vi "Actor Core.vi"(8 "error in":errorcluster, 11 "GPU FFT Calculator in":refnum<class "GPU FFT Calculator.lvclass">) -> (0 "error out":errorcluster, 3 "Actor out":refnum<class "Actor.lvclass">)   [LabVIEW 2020, in "GPU FFT Calculator.lvlib" / "GPU FFT Calculator.lvclass"]
doc: "<p>(<strong>Filename</strong>: <span class=\"dnl\">Actor Framework.lvlib:Actor.lvclass:Actor Core.vi</span>)</p>\n<p>Receives messages to the actor, reacts to them, and initiates any error handling that may shut the actor down.</p>\n<p>Descendant classes may override this VI to append parallel tasks for the actor to complete while it handles messages. Overrides use the <a href=\"nihelplauncher://docs/csh?context=lvcore_glang_udclass\">Call Parent Class Method</a> node.</p>"
uses:
  GPU FFT Calculator.lvclass
  C:/Program Files/National Instruments/LabVIEW 2026/vi.lib/ActorFramework/Actor/Actor.lvclass
  <vilib>/ActorFramework/Actor/Actor.lvclass
  QMH Message.ctl
  <vilib>/Platform/TimedLoop/XDataNode/timing_clust.ctl
  <vilib>/Platform/TimedLoop/XDataNode/nitl_modes.ctl
  <vilib>/Platform/TimedLoop/XDataNode/wakeup.ctl
  GPU FFT Calculator.lvclass/GPU FFT Calculator.ctl
  GPU Device Message.ctl
  <vilib>/Natan Biesmans/G2CPU GPU and CPU HPC Toolkit/ArrayFire Driver/TypeDefs/backend.ctl
  GPU Calculation Message.ctl
  <vilib>/Natan Biesmans/G2CPU GPU and CPU HPC Toolkit/G2CPU Libraries/Async IO/DMA Manager/DMA Manager.lvclass
  <vilib>/Natan Biesmans/G2CPU GPU and CPU HPC Toolkit/G2CPU Libraries/Arrays/1DArray/s16/1D Array s16.lvclass
  C:/Program Files/National Instruments/LabVIEW 2026/vi.lib/Natan Biesmans/G2CPU GPU and CPU HPC Toolkit/G2CPU Libraries/Arrays/Array/Array Prototype.lvclass
  <vilib>/Natan Biesmans/G2CPU GPU and CPU HPC Toolkit/G2CPU Libraries/Arrays/1DArray/f32/1D Array f32.lvclass
  chart zoom.ctl
  GPU Metrics.ctl
  <vilib>/ActorFramework/Actor/Actor.lvclass/Actor.ctl
  <vilib>/ActorFramework/Message Enqueuer/Message Enqueuer.lvclass/Message Enqueuer.ctl
  GPU FFT Calculator Messages/Process Calculation Results Msg/Process Calculation Results Msg.lvclass/Process Calculation Results Msg.ctl
  <vilib>/Natan Biesmans/G2CPU GPU and CPU HPC Toolkit/G2CPU Libraries/Arrays/Array/Array Prototype.lvclass/Array Prototype.ctl
  8c2c1934-b7fc-4e70-9400-bf2723bb4974.vi
  dd08e257-5fd4-41c3-ab12-3278198c71ec.vi
  1389a678-718d-4937-8c80-96463c139bed.vi
  ec50676d-beb5-455b-a2b4-c30064f406c8.vi
  7e026b22-0010-41a1-b2bb-e8234edaae8f.vi
  <vilib>/ActorFramework/Message Enqueuer/Init from Existing Queue.vi
  <vilib>/Natan Biesmans/G2CPU GPU and CPU HPC Toolkit/ArrayFire Driver/VIs/Run as Multi Device.vi
  <vilib>/ActorFramework/Message Enqueuer/Enqueue.vi
  dd08e257-5fd4-41c3-ab12-3278198c71ec.vi/67bb9abe-6be7-467c-be3d-dc59a1f5a88b.vi
  dd08e257-5fd4-41c3-ab12-3278198c71ec.vi/bc198a8f-250c-4fb0-95cf-f9e16e559b40.vi
  dd08e257-5fd4-41c3-ab12-3278198c71ec.vi/206e65cf-1cd8-4fd2-b98d-94b74801007d.vi
  <vilib>/Natan Biesmans/G2CPU GPU and CPU HPC Toolkit/G2CPU Libraries/Arrays/Array/G2CPU Get Array Pointer.vi
  1389a678-718d-4937-8c80-96463c139bed.vi/6197f869-f6d4-49b3-9b2c-cc979b422c2e.vi
  1389a678-718d-4937-8c80-96463c139bed.vi/a7e86dbb-b4c0-485c-89c5-522e60ee265c.vi
  ec50676d-beb5-455b-a2b4-c30064f406c8.vi/ff52a514-0e94-4685-9782-cee11f20a7e4.vi
  ec50676d-beb5-455b-a2b4-c30064f406c8.vi/09f95493-deb6-40ba-ba08-e63bad1f3c71.vi
  7e026b22-0010-41a1-b2bb-e8234edaae8f.vi/7467a0f1-0650-4e63-b635-b3d2b2ec9a4e.vi
  7e026b22-0010-41a1-b2bb-e8234edaae8f.vi/8ee11bc3-5ef5-497e-97f0-8db2b3aaa149.vi
  7e026b22-0010-41a1-b2bb-e8234edaae8f.vi/c7af9698-5e3c-4e11-95da-3024075b67d2.vi
  1389a678-718d-4937-8c80-96463c139bed.vi/6197f869-f6d4-49b3-9b2c-cc979b422c2e.vi/3e802c67-fb96-46a3-ae13-4994a8508b4f.vi
  1389a678-718d-4937-8c80-96463c139bed.vi/6197f869-f6d4-49b3-9b2c-cc979b422c2e.vi/5a50fc67-79e7-4972-80c2-92243cd53dd4.vi
  1389a678-718d-4937-8c80-96463c139bed.vi/6197f869-f6d4-49b3-9b2c-cc979b422c2e.vi/1c928fc9-710a-40e7-8c4f-08a1069452ae.vi
  1389a678-718d-4937-8c80-96463c139bed.vi/a7e86dbb-b4c0-485c-89c5-522e60ee265c.vi/730f6c57-5c0b-4ee9-b61e-75067b25222b.vi
  1389a678-718d-4937-8c80-96463c139bed.vi/a7e86dbb-b4c0-485c-89c5-522e60ee265c.vi/096b8799-7810-404e-baca-ba9279cec4bd.vi
  1389a678-718d-4937-8c80-96463c139bed.vi/a7e86dbb-b4c0-485c-89c5-522e60ee265c.vi/0f1a5a47-bcc5-4796-ac31-8dfcfbc0d7d1.vi
  1389a678-718d-4937-8c80-96463c139bed.vi/a7e86dbb-b4c0-485c-89c5-522e60ee265c.vi/89f12e17-3330-4b72-ad8f-8dd636660732.vi
  1389a678-718d-4937-8c80-96463c139bed.vi/6197f869-f6d4-49b3-9b2c-cc979b422c2e.vi/3e802c67-fb96-46a3-ae13-4994a8508b4f.vi/1b7cf390-2ae0-48f3-9bce-03c57eed6ee8.vi
  GPU FFT Calculator Messages/Process Calculation Results Msg/Process Calculation Results Msg.lvclass
  C:/Program Files/National Instruments/LabVIEW 2026/vi.lib/ActorFramework/Message/Message.lvclass
  <vilib>/Natan Biesmans/G2CPU GPU and CPU HPC Toolkit/G2CPU Libraries/Arrays/1DArray/c32/1D Array c32.lvclass
  <vilib>/Natan Biesmans/G2CPU GPU and CPU HPC Toolkit/G2CPU Libraries/Arrays/2DArray/c32/2D Array c32.lvclass
  <vilib>/Natan Biesmans/G2CPU GPU and CPU HPC Toolkit/G2CPU Libraries/Arrays/2DArray/f32/2D Array f32.lvclass
  <vilib>/Natan Biesmans/G2CPU GPU and CPU HPC Toolkit/ArrayFire Driver/subvi/Error Converter (ErrCode or Status).vi
  <vilib>/Natan Biesmans/G2CPU GPU and CPU HPC Toolkit/G2CPU Libraries/Arrays/Array/G2CPU Set Array Pointer.vi
  <vilib>/Natan Biesmans/G2CPU GPU and CPU HPC Toolkit/G2CPU Libraries/Arrays/SubVI/is 2D.vi
  <vilib>/Natan Biesmans/G2CPU GPU and CPU HPC Toolkit/ArrayFire Driver/VIs/mul.vi
  <vilib>/Natan Biesmans/G2CPU GPU and CPU HPC Toolkit/ArrayFire Driver/VIs/fft inplace.vi
  <vilib>/Natan Biesmans/G2CPU GPU and CPU HPC Toolkit/ArrayFire Driver/VIs/flat.vi
  <vilib>/Natan Biesmans/G2CPU GPU and CPU HPC Toolkit/G2CPU Libraries/Manage Environment/G2CPU Get Backend.vi
  <vilib>/Utility/error.llb/Error Cluster From Error Code.vi
  <vilib>/Natan Biesmans/G2CPU GPU and CPU HPC Toolkit/G2CPU Libraries/Async IO/CUDA Context FGV.vi
  <vilib>/Natan Biesmans/G2CPU GPU and CPU HPC Toolkit/ArrayFire Driver/VIs/copy array.vi
  <vilib>/ActorFramework/Message Priority Queue/Priority Enqueue.vi
  Calculation Worker/Calculation Worker/Calculation Worker.lvclass
  <vilib>/platform/TimedLoop/XDataNode/XDataNode.xnode
  <vilib>/Natan Biesmans/G2CPU GPU and CPU HPC Toolkit/G2CPU Libraries/Arrays/DataTypes/c32/c32.lvclass
  <vilib>/Natan Biesmans/G2CPU GPU and CPU HPC Toolkit/G2CPU Libraries/Arrays/2DArray/2D Array Prototype.lvclass
  <vilib>/Natan Biesmans/G2CPU GPU and CPU HPC Toolkit/G2CPU Libraries/Arrays/Array/Array Prototype.lvclass
  <vilib>/Natan Biesmans/G2CPU GPU and CPU HPC Toolkit/G2CPU Libraries/Arrays/1DArray/1D Array Prototype.lvclass
  <vilib>/Natan Biesmans/G2CPU GPU and CPU HPC Toolkit/G2CPU Libraries/Arrays/DataTypes/f32/f32.lvclass
  <vilib>/ActorFramework/Message Enqueuer/Message Enqueuer.lvclass
  <vilib>/Natan Biesmans/G2CPU GPU and CPU HPC Toolkit/G2CPU Libraries/Manage Environment/G2CPU Manage Environment.lvlib
  <vilib>/Platform/TimedLoop/XDataNode/XDNodeRunTimeDep.lvlib
  <vilib>/Natan Biesmans/G2CPU GPU and CPU HPC Toolkit/ArrayFire Driver/AF.lvlib
  Simple UI/Simple UI/Simple UI.lvclass
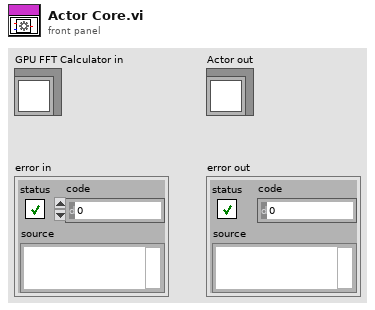
[diagram p1: front panel]
types:
  T1 = typedef "GPU FFT Calculator.lvlib/GPU FFT Calculator.lvclass/QMH Message.ctl" = cluster{"Command":string, "Data":variant}
  T2 = typedef "XDNodeRunTimeDep.lvlib/timing_clust.ctl" = cluster{"Expected End [f-1]":u64, "Actual End [f-1]":u64, "Finished Late? [f-1]":bool, "Expected End [i-1]":u64, "Actual End [i-1]":u64, "Finished Late? [i-1]":bool, "Expected Start [i]":u64, "Actual Start [i]":u64, "Expected Start [f]":u64, "Actual Start [f]":u64, "Source Name":string, "Structure Name":string, "Period":i64, "Deadline":i64, "Offset":i64, "Start":i64, "Priority":i32, "Timeout":i32, "Mode":T3, "Wakeup Reason":T4, "Error":errorcluster, "Source Type":string, "Secondary Source Type":string, "Global End Time":u64, "Global Start Time":u64, "Frame Duration":u64, "Iteration Duration":u64, "Assigned CPU":i32, "I/O Scan Engine Mode":u32}
  T3 = typedef "XDNodeRunTimeDep.lvlib/nitl_modes.ctl" = enum32{"No Change", "Process missed periods, maintain original phase", "Discard missed periods, maintain original phase", "Process missed periods, ignore original phase", "Discard missed periods, ignore original phase"}
  T4 = typedef "XDNodeRunTimeDep.lvlib/wakeup.ctl" = enum32{"Normal", "Aborted", "Asynchronous wakeup", "Timing source error", "Timed loop error", "Timeout"}
  T5 = typedef "GPU FFT Calculator.lvlib/GPU FFT Calculator.lvclass/GPU Device Message.ctl" = cluster{"Backend":T6, "Device ID":i32}
  T6 = typedef "AF.lvlib/backend.ctl" = u32
  T7 = typedef "GPU FFT Calculator.lvlib/GPU FFT Calculator.lvclass/GPU Calculation Message.ctl" = cluster{"FFT Size":u64, "Batch Size":u64, "dt":dbl, "Result Buffer":refnum<data-value>, "gain":dbl, "Zoom Parameters":T8, "Upload DMA Manager":refnum<class "DMA Manager.lvclass">, "Data Buffer":refnum<data-value>, "Data Buffer GPU":refnum<class "1D Array s16.lvclass">, "GPU Metrics":T9, "df":dbl, "f0":dbl, "Zoomed Size":u64, "Result Buffer GPU":refnum<class "1D Array f32.lvclass">, "Start Time":dbl, "Batch Index":i32, "Amount of Batches":i32, "Download DMA Manager":refnum<class "DMA Manager.lvclass">}
  T8 = typedef "Simple UI.lvlib/Simple UI.lvclass/chart zoom.ctl" = cluster{"Override":bool, "f0: ":dbl, "fwidth: ":dbl}
  T9 = typedef "GPU FFT Calculator.lvlib/GPU FFT Calculator.lvclass/GPU Metrics.ctl" = cluster{"Upload Time":dbl, "Algorithm Processing Time":dbl, "Single Trace Size":u64}
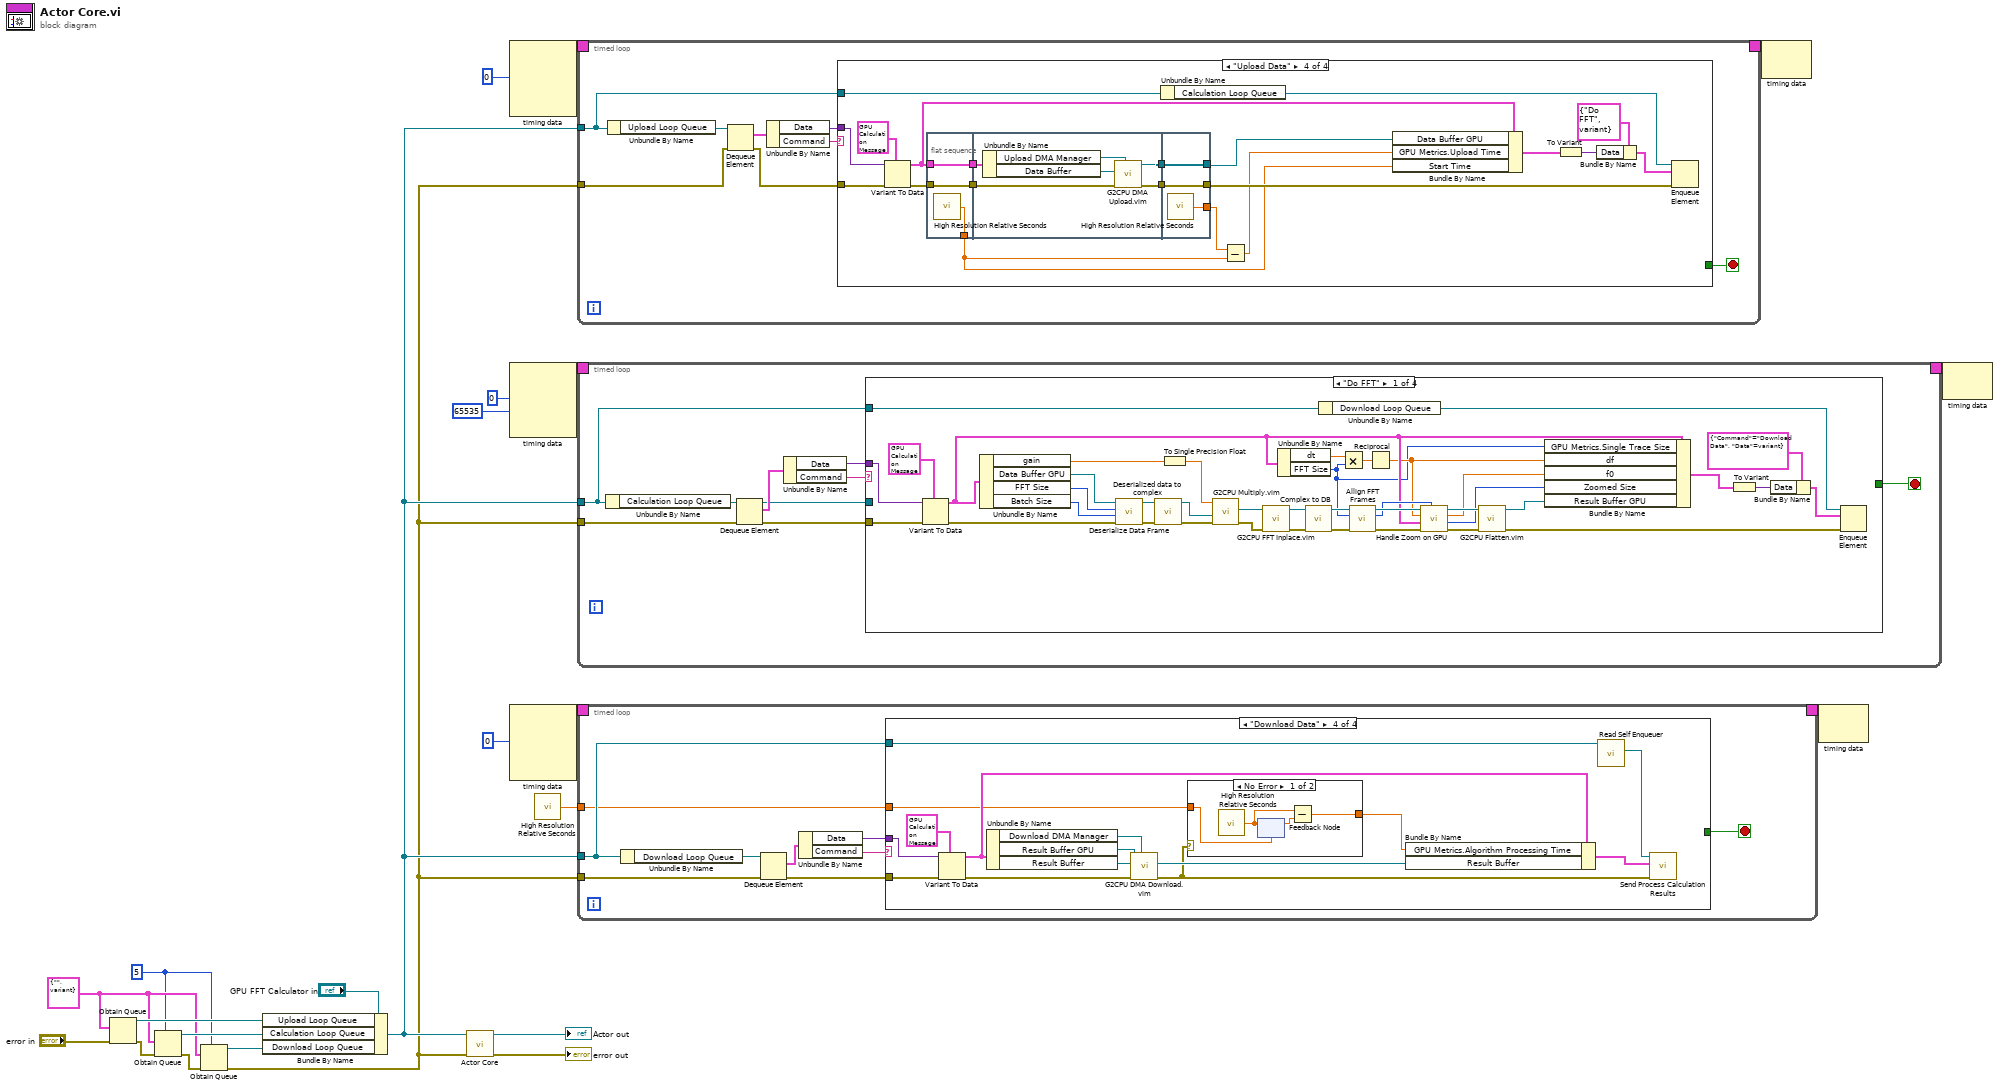
[diagram p0: block diagram]
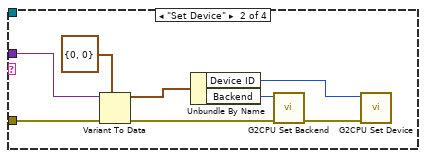
[diagram p3: hidden frame]
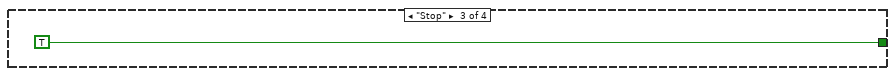
[diagram p4: hidden frame]
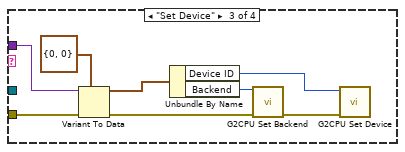
[diagram p6: hidden frame]
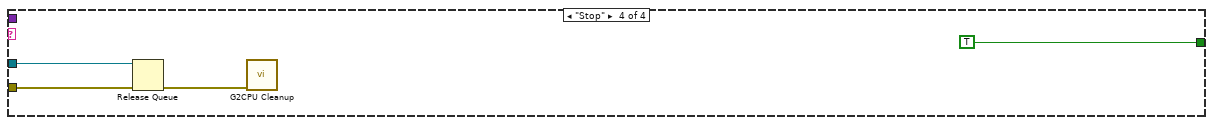
[diagram p7: hidden frame]
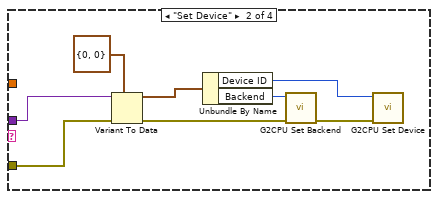
[diagram p9: hidden frame]
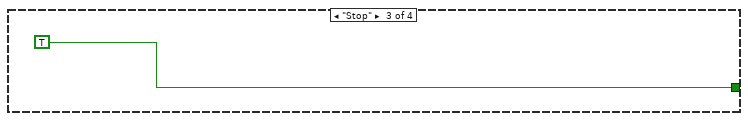
[diagram p10: hidden frame]
diagram:
  w2 = 5 ("max queue size (-1, unlimited)")
  w5 = T1 {"Command"="", "Data"=variant}
  n1 = Obtain Queue(element data type=w5, error in (no error)="error in") -> (queue out=w17:refnum<queue>, error out=w9:errorcluster)  [unwired: 3 in, 1 out]
  n2 = Obtain Queue(max queue size (-1, unlimited)=w2, element data type=w5, error in (no error)=w9) -> (queue out=w8:refnum<queue>, error out=w7:errorcluster)  [unwired: 2 in, 1 out]
  n3 = Obtain Queue(max queue size (-1, unlimited)=w2, element data type=w5, error in (no error)=w7) -> (queue out=w6:refnum<queue>, error out=w4:errorcluster)  [unwired: 2 in, 1 out]
  n4 = Bundle By Name(cluster="GPU FFT Calculator in", "Upload Loop Queue"=w17, "Calculation Loop Queue"=w8, "Download Loop Queue"=w6) -> (w15:refnum<class "GPU FFT Calculator.lvclass">)
  n5 = call-parent "Actor Core.vi"("error in"=w4, "Actor in"=w15) -> ("error out"=→"error out":errorcluster, "Actor out"=→"Actor out":refnum<class "Actor.lvclass">)  [unwired: 8 in]
  n6 = node-c288(i64 0 ("Period")) -> (w14:T2)  [unwired: 3 in]
  n7 = node-c288(i64 0 ("Period"), 65535 ("Priority")) -> (w22:T2)  [unwired: 2 in]
  n8 = node-c288(i64 0 ("Period")) -> (w11:T2)  [unwired: 3 in]
  n9 = call <vilib>:"High Resolution Relative Seconds.vi"() -> ("relative seconds"=w1:dbl)
  n10 = timed-loop {
    timing: w14 -> [_]
    timing-out: [_] -> w13
    tunnel: w15 -> [w25]
    tunnel: w4 -> [w28]
    stop <- w26 stop-if-true
    n11 = Unbundle By Name(w25) -> ("Upload Loop Queue"=w32:refnum<queue>)
    n12 = Dequeue Element(queue=w32, error in (no error)=w28) -> (element=w31:T1, error out=w27:errorcluster)  [unwired: 1 in, 2 out]
    n13 = Unbundle By Name(w31) -> ("Data"=w29:variant, "Command"=w30:string)
    n14 = case shown="\"Upload Data\"" w30 {
      tunnel: w29 -> [_ w34 _ w58]
      tunnel: w27 -> [_ w33 _ w59]
      tunnel: [_ _ TRUE _] -> w26
      tunnel: w25 -> [_ _ _ w51]
      frame "False", Default {
      }
      frame "Set Device" {
        n15 = Variant To Data(error in=w33, type=T5 {"Backend"=0, "Device ID"=0}, Variant=w34) -> (data=w38:T5, error out=w37:errorcluster)
        n16 = Unbundle By Name(w38) -> ("Device ID"=w40:i32, "Backend"=w39:T6)
        n17 = call <vilib>:"G2CPU Set Backend.vi"("error in (no error)"=w37, "Backend"=w39) -> ("error out"=w35:errorcluster)  [unwired: 9 in]
        n18 = call <vilib>:"G2CPU Set Device.vi"("error in (no error)"=w35, "Device ID"=w40) -> ()  [unwired: 9 in, 1 out]
      }
      frame "Stop" {
      }
      frame "Upload Data" {
        n19 = Variant To Data(error in=w59, type=T7 {"FFT Size"=0, "Batch Size"=0, "dt"=0.0, "Result Buffer"=refnum, "gain"=0.0, "Zoom Parameters"={"Override"=FALSE, "f0: "=0.0, "fwidth: "=0.0}, "Upload DMA Manager"=refnum, "Data Buffer"=refnum, "Data Buffer GPU"=refnum, "GPU Metrics"={"Upload Time"=0.0, "Algorithm Processing Time"=0.0, "Single Trace Size"=0}, "df"=0.0, "f0"=0.0, "Zoomed Size"=0, "Result Buffer GPU"=refnum, "Start Time"=0.0, "Batch Index"=0, "Amount of Batches"=0, "Download DMA Manager"=refnum} ("element"), Variant=w58) -> (data=w49:T7, error out=w60:errorcluster)
        n20 = flat-sequence {
          tunnel: w60 -> [w63]
          tunnel: w49 -> [w64]
          tunnel: [w64] -> w55
          tunnel: [w63] -> w54
          tunnel: [w62] -> w42
          tunnel: [w66] -> w57
          tunnel: [w65] -> w56
          tunnel: w55 -> [w70]
          tunnel: w54 -> [w68]
          tunnel: [w72] -> w52
          tunnel: [w73] -> w48
          tunnel: w57 -> [w73]
          tunnel: w56 -> [w72]
          tunnel: [w71] -> w53
          frame #0 {
            n21 = call <vilib>:"High Resolution Relative Seconds.vi"() -> ("relative seconds"=w62:dbl)
          }
          frame #1 {
            n22 = Unbundle By Name(w70) -> ("Upload DMA Manager"=w69:refnum<class "DMA Manager.lvclass">, "Data Buffer"=w67:refnum<data-value>)
            n23 = call "G2CPU DMA Upload.vim"("DMA Manager"=w69, "error in (no error)"=w68, "Data In"=w67) -> ("error out"=w65:errorcluster, "Array out"=w66:refnum<class "1D Array s16.lvclass">)  [unwired: 6 in, 1 out]
          }
          frame #2 {
            n24 = call <vilib>:"High Resolution Relative Seconds.vi"() -> ("relative seconds"=w71:dbl)
          }
        }
        n25 = Unbundle By Name(w51) -> ("Calculation Loop Queue"=w50:refnum<queue>)
        n26 = Subtract(x=w53, y=w42) -> (x-y=w47:dbl)
        n27 = Bundle By Name(cluster=w49, "Data Buffer GPU"=w48, "GPU Metrics.Upload Time"=w47, "Start Time"=w42) -> (w46:T7)
        n28 = To Variant(anything=w46) -> (Variant=w44:variant)
        n29 = Bundle By Name(cluster=T1 {"Command"="Do FFT", "Data"=variant} ("element"), "Data"=w44) -> (w43:T1)
        n30 = Enqueue Element(queue=w50, element=w43, error in (no error)=w52) -> ()  [unwired: 1 in, 3 out]
      }
    }
  }
  n31 = timed-loop {
    timing: w22 -> [_]
    timing-out: [_] -> w21
    tunnel: w15 -> [w77]
    tunnel: w4 -> [w83]
    stop <- w79 stop-if-true
    n32 = Unbundle By Name(w77) -> ("Calculation Loop Queue"=w84:refnum<queue>)
    n33 = Dequeue Element(queue=w84, error in (no error)=w83) -> (queue out=w76:refnum<queue>, element=w78:T1, error out=w81:errorcluster)  [unwired: 1 in, 1 out]
    n34 = Unbundle By Name(w78) -> ("Data"=w80:variant, "Command"=w82:string)
    n35 = case shown="\"Do FFT\"" w82 {
      tunnel: w81 -> [w123 _ w129 w133]
      tunnel: w80 -> [w122 _ w127 _]
      tunnel: [_ _ _ TRUE] -> w79
      tunnel: w76 -> [_ _ _ w134]
      tunnel: w77 -> [w97 _ _ _]
      frame "Do FFT" {
        n36 = Variant To Data(error in=w123, type=T7 {"FFT Size"=0, "Batch Size"=0, "dt"=0.0, "Result Buffer"=refnum, "gain"=0.0, "Zoom Parameters"={"Override"=FALSE, "f0: "=0.0, "fwidth: "=0.0}, "Upload DMA Manager"=refnum, "Data Buffer"=refnum, "Data Buffer GPU"=refnum, "GPU Metrics"={"Upload Time"=0.0, "Algorithm Processing Time"=0.0, "Single Trace Size"=0}, "df"=0.0, "f0"=0.0, "Zoomed Size"=0, "Result Buffer GPU"=refnum, "Start Time"=0.0, "Batch Index"=0, "Amount of Batches"=0, "Download DMA Manager"=refnum} ("element"), Variant=w122) -> (data=w92:T7, error out=w120:errorcluster)
        n37 = Unbundle By Name(w92) -> ("gain"=w100:dbl, "Data Buffer GPU"=w101:refnum<class "1D Array s16.lvclass">, "FFT Size"=w117:u64, "Batch Size"=w116:u64)
        n38 = call "Deserialize Data Frame.vi"("error in (no error)"=w120, "Batch Size"=w116, "FFT Size"=w117, "Serial Data In"=w101) -> ("error out"=w115:errorcluster, "Deserialized Data Out"=w114:refnum<class "3D Array s16.lvclass">)  [unwired: 6 in]
        n39 = call "Deserialized data to complex.vi"("error in (no error)"=w115, "Deserialized Data In"=w114) -> ("error out"=w113:errorcluster, "Complex Data Out"=w112:refnum<class "2D Array c32.lvclass">)  [unwired: 8 in]
        n40 = To Single Precision Float(number=w100) -> (single precision float=w109:sgl)
        n41 = call "G2CPU Multiply.vim"("error in (no error)"=w113, "Array rhs"=w112, "Array lhs"=w109) -> ("error out"=w107:errorcluster, "Array Result"=w108:refnum<class "2D Array c32.lvclass">)  [unwired: 7 in]
        n42 = call "G2CPU FFT Inplace.vim"("error in (no error)"=w107, "Array Signal"=w108) -> ("error out"=w111:errorcluster, "Array out"=w110:refnum<class "2D Array c32.lvclass">)  [unwired: 8 in]
        n43 = Unbundle By Name(w92) -> ("dt"=w118:dbl, "FFT Size"=w85:u64)
        n44 = call "Complex to DB.vi"("error in (no error)"=w111, "Complex Data In"=w110) -> ("error out"=w102:errorcluster, "Amplitude dB Out"=w106:refnum<class "2D Array f32.lvclass">)  [unwired: 8 in]
        n45 = Unbundle By Name(w97) -> ("Download Loop Queue"=w93:refnum<queue>)
        n46 = Multiply(x=w118, y=w85) -> (x*y=w119:dbl)
        n47 = call "Allign FFT Frames.vi"("error in (no error)"=w102, "FFT Size"=w85, "Unalligned FFT Amplitudes"=w106) -> ("error out"=w104:errorcluster, "FFT Size / 2"=w103:u64, "Unalligned FFT Amplitudes"=w105:refnum<class "2D Array f32.lvclass">)  [unwired: 6 in]
        n48 = Reciprocal(x=w119) -> (1/x=w91:dbl)
        n49 = call "Handle Zoom on GPU.vi"("FFT Size / 2 in"=w103, "error in (no error)"=w104, "element"=w92, "df"=w91, "Unzoomed Data In"=w105) -> ("error out"=w98:errorcluster, "Zoomed Size"=w89:u64, "f0:"=w90:dbl, "Zoomed Data Out"=w99:refnum<class "2D Array f32.lvclass">)  [unwired: 3 in]
        n50 = call "G2CPU Flatten.vim"("error in (no error)"=w98, "Array In"=w99) -> ("error out"=w86:errorcluster, "Array out"=w88:refnum<class "1D Array f32.lvclass">)  [unwired: 8 in]
        n51 = Bundle By Name(cluster=w92, "GPU Metrics.Single Trace Size"=w85, "df"=w91, "f0"=w90, "Zoomed Size"=w89, "Result Buffer GPU"=w88) -> (w87:T7)
        n52 = To Variant(anything=w87) -> (Variant=w95:variant)
        n53 = Bundle By Name(cluster=T1 {"Command"="Download Data", "Data"=variant} ("element"), "Data"=w95) -> (w96:T1)
        n54 = Enqueue Element(queue=w93, element=w96, error in (no error)=w86) -> ()  [unwired: 1 in, 3 out]
      }
      frame Default {
      }
      frame "Set Device" {
        n55 = Variant To Data(error in=w129, type=T5 {"Backend"=0, "Device ID"=0}, Variant=w127) -> (data=w126:T5, error out=w128:errorcluster)
        n56 = Unbundle By Name(w126) -> ("Device ID"=w124:i32, "Backend"=w125:T6)
        n57 = call <vilib>:"G2CPU Set Backend.vi"("error in (no error)"=w128, "Backend"=w125) -> ("error out"=w131:errorcluster)  [unwired: 9 in]
        n58 = call <vilib>:"G2CPU Set Device.vi"("error in (no error)"=w131, "Device ID"=w124) -> ()  [unwired: 9 in, 1 out]
      }
      frame "Stop" {
        n59 = Release Queue(queue=w134, error in (no error)=w133) -> (error out=w132:errorcluster)  [unwired: 1 in, 2 out]
        n60 = call <vilib>:"G2CPU Cleanup.vi"("error in (no error)"=w132) -> ()  [unwired: 10 in, 1 out]
      }
    }
  }
  n61 = timed-loop {
    timing: w11 -> [_]
    timing-out: [_] -> w10
    tunnel: w15 -> [w139]
    tunnel: w4 -> [w141]
    tunnel: w1 -> [w138]
    stop <- w140 stop-if-true
    n62 = Unbundle By Name(w139) -> ("Download Loop Queue"=w142:refnum<queue>)
    n63 = Dequeue Element(queue=w142, error in (no error)=w141) -> (element=w143:T1, error out=w146:errorcluster)  [unwired: 1 in, 2 out]
    n64 = Unbundle By Name(w143) -> ("Data"=w145:variant, "Command"=w144:string)
    n65 = case shown="\"Download Data\"" w144 {
      tunnel: w145 -> [_ w148 _ w164]
      tunnel: w146 -> [_ w147 _ w165]
      tunnel: [_ _ TRUE _] -> w140
      tunnel: w139 -> [_ _ _ w166]
      tunnel: w138 -> [_ _ _ w157]
      frame "False", Default {
      }
      frame "Set Device" {
        n66 = Variant To Data(error in=w147, type=T5 {"Backend"=0, "Device ID"=0}, Variant=w148) -> (data=w152:T5, error out=w151:errorcluster)
        n67 = Unbundle By Name(w152) -> ("Device ID"=w154:i32, "Backend"=w153:T6)
        n68 = call <vilib>:"G2CPU Set Backend.vi"("error in (no error)"=w151, "Backend"=w153) -> ("error out"=w149:errorcluster)  [unwired: 9 in]
        n69 = call <vilib>:"G2CPU Set Device.vi"("error in (no error)"=w149, "Device ID"=w154) -> ()  [unwired: 9 in, 1 out]
      }
      frame "Stop" {
      }
      frame "Download Data" {
        n70 = Variant To Data(error in=w165, type=T7 {"FFT Size"=0, "Batch Size"=0, "dt"=0.0, "Result Buffer"=refnum, "gain"=0.0, "Zoom Parameters"={"Override"=FALSE, "f0: "=0.0, "fwidth: "=0.0}, "Upload DMA Manager"=refnum, "Data Buffer"=refnum, "Data Buffer GPU"=refnum, "GPU Metrics"={"Upload Time"=0.0, "Algorithm Processing Time"=0.0, "Single Trace Size"=0}, "df"=0.0, "f0"=0.0, "Zoomed Size"=0, "Result Buffer GPU"=refnum, "Start Time"=0.0, "Batch Index"=0, "Amount of Batches"=0, "Download DMA Manager"=refnum} ("element"), Variant=w164) -> (data=w162:T7, error out=w169:errorcluster)
        n71 = Unbundle By Name(w162) -> ("Download DMA Manager"=w160:refnum<class "DMA Manager.lvclass">, "Result Buffer GPU"=w159:refnum<class "1D Array f32.lvclass">, "Result Buffer"=w161:refnum<data-value>)
        n72 = call "G2CPU DMA Download.vim"("DMA Manager"=w160, "error in (no error)"=w169, "Data In"=w161, "GPU CUDA Array In"=w159) -> ("error out"=w158:errorcluster, "Data Out"=w163:refnum<data-value>)  [unwired: 5 in, 1 out]
        n73 = case shown="No Error" w158 {
          tunnel: w157 -> [w171 _]
          tunnel: [w172 _] -> w156
          frame No Error {
            n74 = call <vilib>:"High Resolution Relative Seconds.vi"() -> ("relative seconds"=w173:dbl)
            n75 = feedback-in #1(w173) -> ()
            n76 = feedback #1(w171) -> (w174:dbl)
            n77 = Subtract(x=w173, y=w174) -> (x-y=w172:dbl)
          }
          frame Error {
          }
        }
        n78 = Bundle By Name(cluster=w162, "GPU Metrics.Algorithm Processing Time"=w156, "Result Buffer"=w163) -> (w168:T7)
        n79 = call <vilib>:"Read Self Enqueuer.vi"("Actor"=w166) -> ("Self Enqueuer"=w167:refnum<class "Message Enqueuer.lvclass">)  [unwired: 10 in]
        n80 = call "Send Process Calculation Results.vi"("error in (no error)"=w158, "GPU Calculation Results"=w168, "Message Enqueuer"=w167) -> ()  [unwired: 7 in, 2 out]
      }
    }
  }
  n81 = node-c288(w13) -> ()  [unwired: 1 out]
  n82 = node-c288(w10) -> ()  [unwired: 1 out]
  n83 = node-c288(w21) -> ()  [unwired: 1 out]
